vi "Disconnect (SubVI).vi"(8 "error in (no error)":errorcluster, 11 "paramUnicornIn":T1) -> (0 "error out":errorcluster, 3 "paramUnicornIn 2":T1)   [LabVIEW 2017, in "LV_Unicorn.lvlib"]
uses:
  LV_Unicorn.lvlib
  Control/unicorn_Param.ctl
  Control/unicorn_conn.ctl
  Control/unicorn_JSON.ctl
  Control/unicorn_ParamInt.ctl
  Control/unicorn_Telemetry.ctl
  Control/unicorn_Table.ctl
  Control/unicorn_ParamFloat.ctl
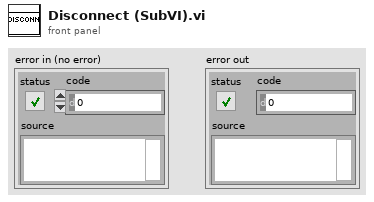
[diagram p1: front panel]
types:
  T1 = typedef "LV_Unicorn.lvlib/unicorn_Param.ctl" = cluster{"conParam":T2, "Param":T3}
  T2 = typedef "LV_Unicorn.lvlib/unicorn_conn.ctl" = cluster{"ReadIntParam":bool, "ReadDescrParam":bool, "ReadFloatParam":bool, "debug":bool, "ReadJSON":bool, "IP_address":string, "N_attempts":i32, "type_con":enum16{"Serial", "TCP"}, "MB_address":i32, "VISA":refnum<visa-resource-name>, "connection ID":refnum<k5>, "nameDevices":string, "timeout":i32, "port":u16, "type_version":string, "baud_rate":u32, "VersionControl":bool, "TCP_conn":bool, "WindowSize":i32}
  T3 = typedef "LV_Unicorn.lvlib/unicorn_JSON.ctl" = cluster{"NumParam":cluster{"NTelem":i32, "NInt":i32, "NFloat":i32, "NTable":i32}, "ParamInt":T4, "Telemetry":T5, "Table":T6, "ParamFloat":T7}
  T4 = typedef "LV_Unicorn.lvlib/unicorn_ParamInt.ctl" = cluster{"ID":string, "Num":i32, "Name":string, "Type":string, "Enum":string, "Desc":string, "Unit":string, "Access":string, "FormatStr":string, "Min":i32, "Max":i32}[]
  T5 = typedef "LV_Unicorn.lvlib/unicorn_Telemetry.ctl" = cluster{"ID":string, "Num":i32, "Name":string, "Desc":string, "Unit":string, "FormatStr":string, "Min":i32, "Max":i32}[]
  T6 = typedef "LV_Unicorn.lvlib/unicorn_Table.ctl" = cluster{"Num":i32, "Access":string, "ColumnCount":i32, "NeedParamPrepare":bool, "Columns":cluster{"Column":i32, "Desc":string, "Name":string}[], "DataType":string, "FormatStr":string, "ID":string, "Name":string, "RowCount":i32, "Rows":cluster{"Desc":string, "ID":string, "Max":i32, "Min":i32, "Name":string, "Row":i32, "Unit":string}[], "Type":string}[]
  T7 = typedef "LV_Unicorn.lvlib/unicorn_ParamFloat.ctl" = cluster{"ID":string, "Num":i32, "Name":string, "Type":string, "Enum":string, "Desc":string, "Unit":string, "Access":string, "FormatStr":string, "Min":sgl, "Max":sgl}[]
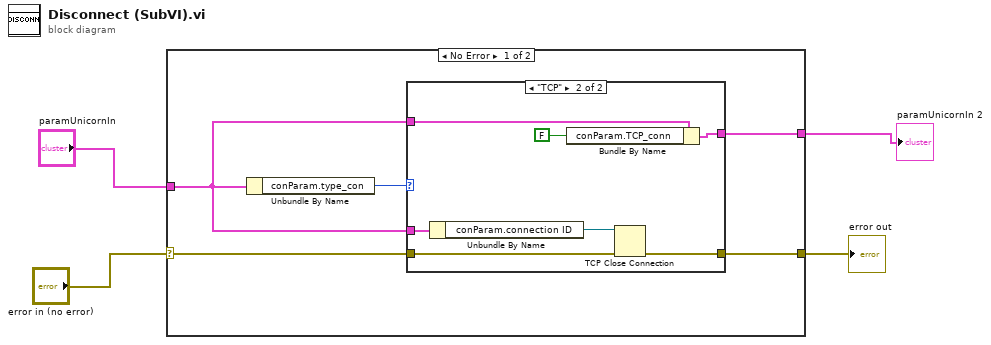
[diagram p0: block diagram]
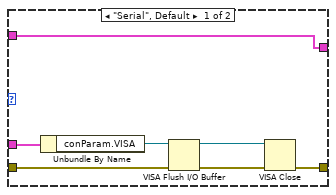
[diagram p2: hidden frame]
diagram:
  n1 = case shown="No Error" "error in (no error)" {
    selector: "error in (no error)" -> [w8 w25]
    tunnel: "paramUnicornIn" -> [w5 w24]
    tunnel: [w7 w25] -> w4
    tunnel: [w6 w24] -> w1
    frame No Error {
      n2 = Unbundle By Name(w5) -> ("conParam.type_con"=w9:enum16{"Serial", "TCP"})
      n3 = case shown="\"TCP\"" w9 {
        tunnel: w8 -> [w15 w23]
        tunnel: [w14 w22] -> w7
        tunnel: w5 -> [w12 w21]
        tunnel: w5 -> [w10 w19]
        tunnel: [w10 w17] -> w6
        frame "Serial", Default {
          n4 = Unbundle By Name(w12) -> ("conParam.VISA"=w11:refnum<visa-resource-name>)
          n5 = VISA Flush I/O Buffer(VISA resource name=w11, error in (no error)=w15) -> (VISA resource name out=w13:refnum<visa-resource-name>, error out=w16:errorcluster)  [unwired: 1 in]
          n6 = VISA Close(VISA resource name=w13, error in (no error)=w16) -> (error out=w14:errorcluster)
        }
        frame "TCP" {
          n7 = Unbundle By Name(w21) -> ("conParam.connection ID"=w20:refnum<k5>)
          n8 = Bundle By Name(cluster=w19, "conParam.TCP_conn"=FALSE) -> (w17:T1)
          n9 = TCP Close Connection(connection ID=w20, error in (no error)=w23) -> (error out=w22:errorcluster)  [unwired: 1 in, 1 out]
        }
      }
    }
    frame Error {
    }
  }
  "error out" <- w4
  "paramUnicornIn 2" <- w1
